vi "Forward Pass [Gate] (LSTM).vi"(0 "x[t]":T1=[[0.0], [1.0], [0.0]], 2 "h[t-1]":T1=[[0.9], [0.1]], 4 "c[t-1]":T1=[[0.9], [0.1]], 5 "params":cluster{"Wxq":T1, "Whq":T1, "Wcq":T1, "bq":T1}={"Wxq"=[[0.57813, 2.5697, -0.0219857], [-2.4696, -0.172737, 2.44961362]], "Whq"=[[-1.39960002, 0.96174453], [0.36456552, -0.47706397]], "Wcq"=[[-0.6486, 0.76469], [-1.77899, 0.38803572]], "bq"=[[0.5353143], [-1.98598657]]}, 7 "Activation":enum16{"sigmoid", "tanh", "ReLU", "Identity"}(ring)) -> (16 "Vector":T1=[[0.11924558384048108], [0.9291561164037933]])   [LabVIEW 2014]
uses:
  <vilib>/Analysis/Matrix/Datatypes/RealMatrix.ctl
  <vilib>/Analysis/baseanly.llb/Real A x B.vi
  <vilib>/Analysis/Matrix/Numeric/Add/Add - RM,RM.vi
  <vilib>/Analysis/NI_AALBase.lvlib
  <vilib>/Analysis/Matrix/NI_Matrix.lvlib
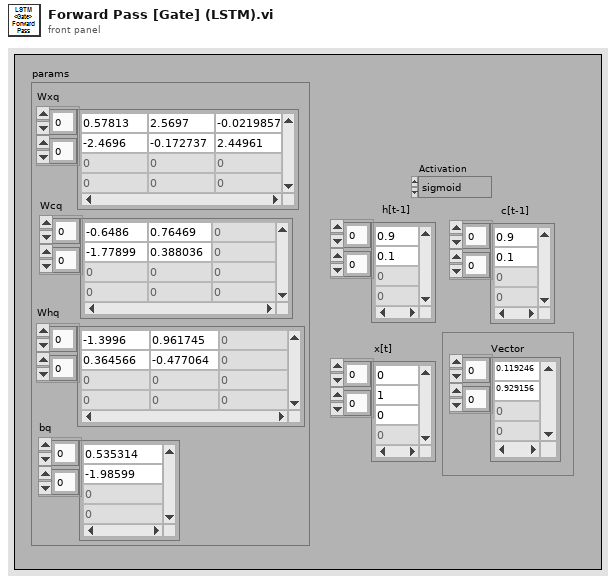
[diagram p1: front panel]
types:
  T1 = typedef "NI_Matrix.lvlib/RealMatrix.ctl" = dbl[][]
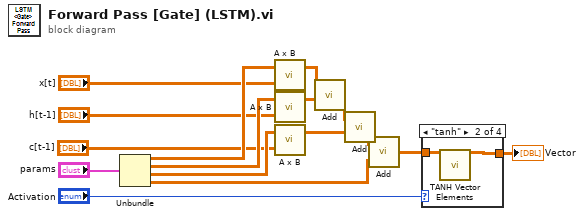
[diagram p0: block diagram]
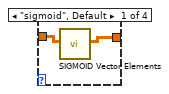
[diagram p2: hidden frame]
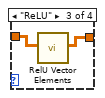
[diagram p3: hidden frame]
diagram:
  n1 = Unbundle("params") -> ("Wxq"=w8:T1, "Whq"=w9:T1, "Wcq"=w10:T1, "bq"=w11:T1)
  n2 = call-poly <vilib>:"A x B.vi"("B"="x[t]", "A"=w8) -> ("A x B"=w16:T1)  [unwired: 1 out]
  n3 = call-poly <vilib>:"A x B.vi"("B"="h[t-1]", "A"=w9) -> ("A x B"=w15:T1)  [unwired: 1 out]
  n4 = call-poly <vilib>:"A x B.vi"("B"="c[t-1]", "A"=w10) -> ("A x B"=w13:T1)  [unwired: 1 out]
  n5 = call-poly <vilib>:"Add.vi"("Real Matrix B"=w15, "Real Matrix A"=w16) -> ("A + B"=w14:T1)
  n6 = call-poly <vilib>:"Add.vi"("Real Matrix B"=w13, "Real Matrix A"=w14) -> ("A + B"=w7:T1)
  n7 = call-poly <vilib>:"Add.vi"("Real Matrix B"=w11, "Real Matrix A"=w7) -> ("A + B"=w3:T1)
  n8 = case shown="\"tanh\"" "Activation" {
    tunnel: w3 -> [w18 w20 w22 w23]
    tunnel: [w17 w19 w21 w23] -> w2
    frame "sigmoid", Default {
      n9 = call "SIGMOID Vector Elements.vi"("X"=w18) -> ("sigmoid(X)"=w17:T1)  [unwired: 18 in]
    }
    frame "tanh" {
      n10 = call "TANH Vector Elements.vi"("X"=w20) -> ("tanh(X)"=w19:T1)  [unwired: 18 in]
    }
    frame "ReLU" {
      n11 = call "RelU Vector Elements.vi"("X"=w22) -> ("RelU(X)"=w21:T1)  [unwired: 18 in]
    }
    frame "Identity" {
    }
  }
  "Vector" <- w2
